vi "Write str to xls File.vi"(4 "Flush interval (s)":dbl=60.0 format="%.2f", 6 "transpose? (no:F)":bool, 7 "format (%.s)":string="%s", 8 "error in (no error)":errorcluster, 9 "2D data":string[][](array[string]), 10 "1D data":string[](array[string]), 11 "refnum":refnum<file>) -> (0 "error out":errorcluster, 3 "dup refnum":refnum<file>)   [LabVIEW 2015]
panel:
  out "spreadsheet string":string
  out "bad file ref":bool
  in  "delimiter (Tab)":string="\t"
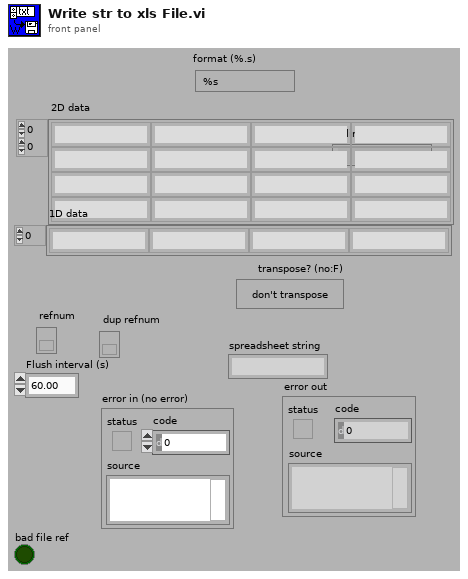
[diagram p1: front panel]
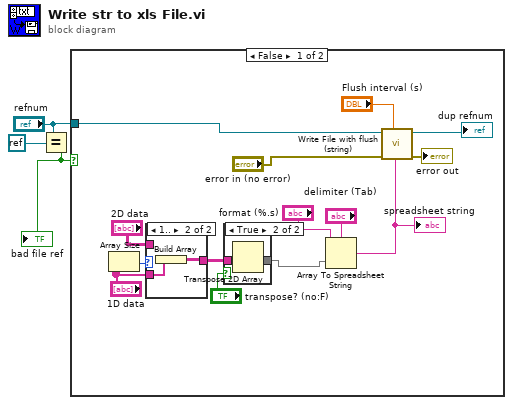
[diagram p0: block diagram]
diagram:
  n1 = Equal?(x="refnum", y=refnum<k0> refnum) -> (x = y?=w1:bool)
  "bad file ref" <- w1
  n2 = case shown="False" w1 {
    tunnel: "refnum" -> [w10 _]
    frame False {
      n3 = Array Size(array="1D data") -> (size(s)=w17:i32)
      n4 = case shown="1.." w17 {
        tunnel: "1D data" -> [_ w23]
        tunnel: [w21 w22] -> w13
        tunnel: "2D data" -> [w21 _]
        frame ..0 {
          # "1D array is empty"
        }
        frame 1.. {
          n5 = Build Array(w23) -> (w22:string[][])
        }
      }
      n6 = case shown="True" "transpose? (no:F)" {
        tunnel: [w18 w20] -> w5
        tunnel: w13 -> [w18 w19]
        frame False {
        }
        frame True {
          n7 = Transpose 2D Array(2D array=w19) -> (transposed array=w20:string[][])
        }
      }
      n8 = Array To Spreadsheet String(delimiter (Tab)="delimiter (Tab)", array=w5, 3:"format (%.s)") -> (spreadsheet string=w6:string)
      "spreadsheet string" <- w6
      n9 = call "Write File with flush (string).vi"("string"=w6, "Flush interval (s)"="Flush interval (s)", "error in (no error)"="error in (no error)", "refnum"=w10) -> ("error out"=→"error out":errorcluster, "dup refnum"=→"dup refnum":refnum<file>)  [unwired: 4 in, 1 out]
    }
    frame True {
    }
  }
